vi "LIN Graph.vi"   [LabVIEW 2020, in "Linearisierung v2.lvlib"]
uses:
  Linearisierung v2.lvlib
  SpanEinstellungen/Aktion FGV SpanEinstellungen.ctl
  SpanEinstellungen/Aktion FGV Spans abarbeiten.ctl
  f64b9011-796f-4909-a89d-b7e0acf8c31b.vi
  Protokoll/Protokoll.lvlib
  Allgemein/allgemeine Sub-VIs.lvlib
  SpanEinstellungen/SpanEinstellungen.lvlib
types:
  T1 = typedef "Linearisierung v2.lvlib/SpanEinstellungen.lvlib/Aktion FGV Spans abarbeiten.ctl" = enum16{"lesen", "idle", "start", "next", "comp", "init", "running", "abort"}
  T2 = typedef "Linearisierung v2.lvlib/SpanEinstellungen.lvlib/Aktion FGV SpanEinstellungen.ctl" = enum16{"lesen", "schreiben", "laden", "speichern", "RegisterRef", "automatisch", "init", "PDF Params", "Punkte umkehren"}
  T3 = cluster{"Dieses VI":refnum<vi>, "Cluster (Eingang)":refnum<vi>, "Graphik (Eingang)":refnum<vi>, "Clear (Eingang)":refnum<vi>}
  T4 = typedef "System Einstellungen V2.lvlib/Konfig Gasflasche.ctl" = bool
  T5 = typedef "Linearisierung v2.lvlib/SpanEinstellungen.lvlib/SpanInletCluster.ctl" = cluster{"Span Inlet Active":T4, "Analysator":T6, "Konfig Gasflasche":T4, "Gasflasche":T7, "Gasflaschen Nr.:":string, "Ablaufdatum":timestamp, "Komponenten":T8, "Zeitdauer Stufen":sgl, "Max Fehler":sgl, "Anzahl Stufen":sgl, "Trägergas":T12, "zusätzliche Zeitdauer Erster Punkt":sgl}
  T6 = typedef "System Einstellungen V2.lvlib/Analysatoren.ctl" = string
  T7 = typedef "System Einstellungen V2.lvlib/Gasflasche Auswahl.ctl" = u16
  T8 = typedef "Linearisierung v2.lvlib/SpanEinstellungen.lvlib/Komponentencluster mit Formel.ctl" = cluster{"Komponente 1":T9, "Komponente 2":T9, "Komponente 3":T9, "Komponente 4":T9, "Komponente 5":T9}
  T9 = typedef "Linearisierung v2.lvlib/SpanEinstellungen.lvlib/Komponentenauswahl mit Formel.ctl" = cluster{"Komponente:":u16, "Summenformel":T10, "Konzentration IST":dbl, "Einheit":T11, "Genauigkeit":dbl}
  T10 = typedef "String - Eingabefeld.ctl" = string
  T11 = typedef "Linearisierung v2.lvlib/SpanEinstellungen.lvlib/Einheit.ctl" = enum16{"ppm", "%"}
  T12 = typedef "System Einstellungen V2.lvlib/Traegergas.ctl" = string
  T13 = cluster{"Array out[0]":u16, "Array out[1]":u16, "Array out[2]":u16, "Array out[3]":u16, "Array out[4]":u16, "Array out[5]":u16}
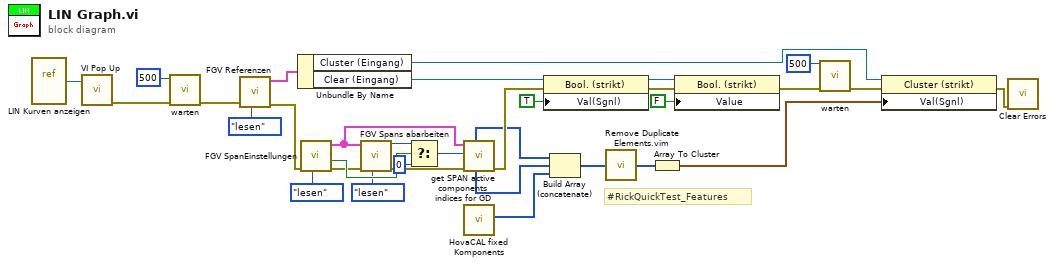
[diagram p0: block diagram]
diagram:
  # "#RickQuickTest_Features"
  n1 = vi-ref "LIN Kurven anzeigen.vi"() -> (w13:refnum<vi>)
  n2 = call "VI Pop Up.vi"("VI Referenz"=w13) -> ("error out"=w7:errorcluster)  [unwired: 10 in]
  n3 = call "warten.vi"("error in (no error)"=w7, "Zu wartende ms"=u32 500) -> ("error out"=w6:errorcluster)  [unwired: 8 in, 1 out]
  n4 = call "FGV Referenzen.vi"("Aktikon"=enum16{"lesen", "schreiben"}."lesen", "error in (no error)"=w6) -> ("error out"=w22:errorcluster, "Referenzen Cluster out"=w14:T3)  [unwired: 7 in]
  n5 = Unbundle By Name(w14) -> ("Cluster (Eingang)"=w1:refnum<vi>, "Clear (Eingang)"=w2:refnum<vi>)
  n6 = call "FGV SpanEinstellungen.vi"("Aktion"=Aktion_FGV_SpanEinstellungen."lesen", "error in (no error)"=w22) -> ("error out"=w20:errorcluster, "automatisch out"=w25:T4, "SpanInletClusterArray out"=w19:T5[])  [unwired: 5 in, 2 out]
  n7 = call "FGV Spans abarbeiten.vi"("Aktion"=Aktion_FGV_Spans_abarbeiten."lesen", "error in (no error)"=w20, "SpanInletClusterArray in"=w19) -> ("error out"=w21:errorcluster, "active SPAN Idx out"=w27:i32)  [unwired: 3 in, 4 out]
  n8 = Select(t=w27, s=w25, f=0 ("active SPAN Idx out")) -> (s? t:f=w28:i32)
  n9 = call "get SPAN active components indices for GD.vi"("error in (no error)"=w21, "SPAN Idx"=w28, "SpanInletClusterArray in"=w19) -> ("error out"=w33:errorcluster, "aktive Komponenten additional"=w15:u16[], "aktive Komponenten GD"=w16:u16[])  [unwired: 1 in, 5 out]
  n10 = call "HovaCAL fixed Komponents.vi"() -> ("MFV Komponente fix out"=w11:u16[])  [unwired: 10 in, 1 out]
  n11 = property class="Bool. (strikt)"(reference=w2, error in=w33, "Val(Sgnl)"=TRUE ("Wert (signalisierend)")) -> (reference out=w31:refnum<vi>, error out=w32:errorcluster)
  n12 = Build Array (concatenate)(w16, w15, w11) -> (w10:u16[])
  n13 = call "Remove Duplicate Elements.vim"("Array in"=w10) -> ("Array out"=w9:u16[])
  n14 = Array To Cluster(array=w9) -> (cluster=w24:T13)
  n15 = property class="Bool. (strikt)"(reference=w31, error in=w32, "Value"=FALSE ("Wert")) -> (error out=w4:errorcluster)  [unwired: 1 out]
  n16 = call "warten.vi"("error in (no error)"=w4, "Zu wartende ms"=u32 500) -> ("error out"=w3:errorcluster)  [unwired: 8 in, 1 out]
  n17 = property class="Cluster (strikt)"(reference=w1, error in=w3, "Val(Sgnl)"=w24) -> (error out=w23:errorcluster)  [unwired: 1 out]
  n18 = call <vilib>:"Clear Errors.vi"("error in (no error)"=w23) -> ()  [unwired: 5 in, 2 out]
